vi "Read Test Method Names.vi"(8 "error in (no error)":errorcluster, 10 "Test Case":string, 11 "Test Case Finder In":refnum<class "Test Finder.lvclass">) -> (0 "error out":errorcluster, 2 "Names":T1(array[cluster]), 3 "Test Case Finder Out":refnum<class "Test Finder.lvclass">)   [LabVIEW 2020, in "Test Finder.lvclass"]
uses:
  Test Finder.lvclass
  Test Finder.lvclass/Test Finder.ctl
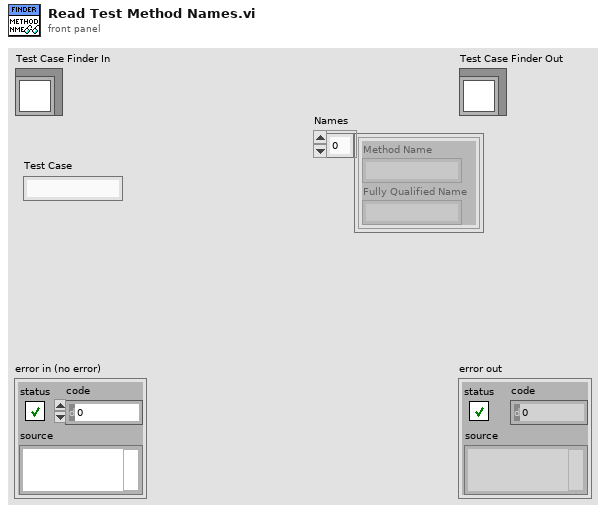
[diagram p1: front panel]
types:
  T1 = cluster{"Method Name":string, "Fully Qualified Name":string}[]
  T2 = map{string, cluster{"Inherited Methods":map{string, path}, "Owned Methods":map{string, path}}}
  T3 = cluster{"Method Name":string, "Fully Qualified Name":string}
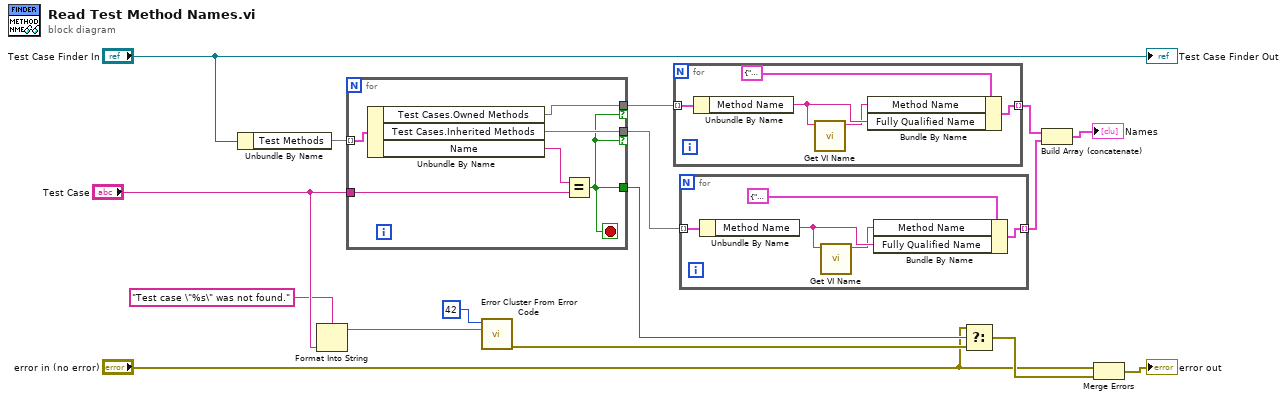
[diagram p0: block diagram]
diagram:
  n1 = Unbundle By Name("Test Case Finder In") -> ("Test Methods"=w15:T2)
  n2 = Format Into String(format string="Test case \"%s\" was not found.", "Test Case") -> (resulting string=w7:string)  [unwired: 2 in, 1 out]
  n3 = for {
    tunnel: w15 -> [w22] mode=indexing
    tunnel: [w19] -> w6 if=w17
    tunnel: "Test Case" -> [w20]
    tunnel: [w17] -> w14
    tunnel: [w18] -> w4 if=w17
    stop <- w17 stop-if-true
    n4 = Unbundle By Name(w22) -> ("Test Cases.Owned Methods"=w18:map{string, path}, "Test Cases.Inherited Methods"=w19:map{string, path}, "Name"=w21:string)
    n5 = Equal?(x=w21, y=w20) -> (x = y?=w17:bool)
  }
  n6 = call <vilib>:"Error Cluster From Error Code.vi"("error message (\"\")"=w7, "error code (0)"=42) -> ("error out"=w11:errorcluster)  [unwired: 7 in]
  n7 = for {
    tunnel: [w23] -> w3 mode=indexing
    tunnel: w4 -> [w27] mode=indexing
    n8 = Unbundle By Name(w27) -> ("Method Name"=w25:string)
    n9 = call "Get VI Name.vi"("Fully Qualified VI name"=w25) -> ("VI Name"=w24:string)  [unwired: 9 in, 1 out]
    n10 = Bundle By Name(cluster=T3 {"Method Name"="", "Fully Qualified Name"=""} ("Names"), "Method Name"=w24, "Fully Qualified Name"=w25) -> (w23:T3)
  }
  n11 = for {
    tunnel: [w28] -> w2 mode=indexing
    tunnel: w6 -> [w32] mode=indexing
    n12 = Unbundle By Name(w32) -> ("Method Name"=w30:string)
    n13 = call "Get VI Name.vi"("Fully Qualified VI name"=w30) -> ("VI Name"=w29:string)  [unwired: 9 in, 1 out]
    n14 = Bundle By Name(cluster=T3 {"Method Name"="", "Fully Qualified Name"=""} ("Names"), "Method Name"=w29, "Fully Qualified Name"=w30) -> (w28:T3)
  }
  n15 = Select(t="error in (no error)", s=w14, f=w11) -> (s? t:f=w12:errorcluster)
  n16 = Build Array (concatenate)(w3, w2) -> (→"Names":T1)
  n17 = Merge Errors("error in (no error)", w12) -> (→"error out":errorcluster)
  "Test Case Finder Out" <- "Test Case Finder In"
